vi "DB Update.vi"(8 "error in (no error)":errorcluster, 10 "SQL query":string, 11 "Database in":refnum<class "MYSQL Database.lvclass">) -> (0 "error out":errorcluster, 3 "Database out":refnum<class "MYSQL Database.lvclass">)   [LabVIEW 2023, in "HardwareAbstractionLayer_LVOOP.lvlib" / "MYSQL Database.lvclass"]
uses:
  MYSQL Database.lvclass
  MYSQL Database.lvclass/MYSQL Database.ctl
  <vilib>/addons/database/Connection.llb/Conn Execute.vi
  <vilib>/addons/database/Recordset.llb/Rec Destroy - Connection.vi
  <vilib>/addons/database/NI_Database_API.lvlib
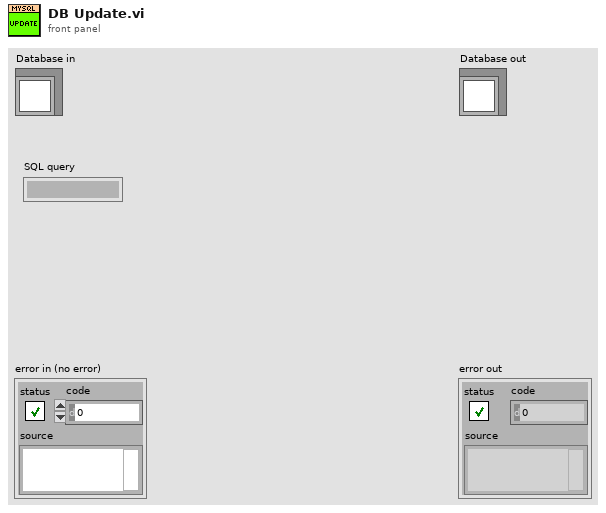
[diagram p1: front panel]
types:
  T1 = typedef "NI_Database_API.lvlib/Conn ObjectReference.ctl" = refnum<k1>
  T2 = typedef "NI_Database_API.lvlib/Rec ObjectReference.ctl" = refnum<k1>
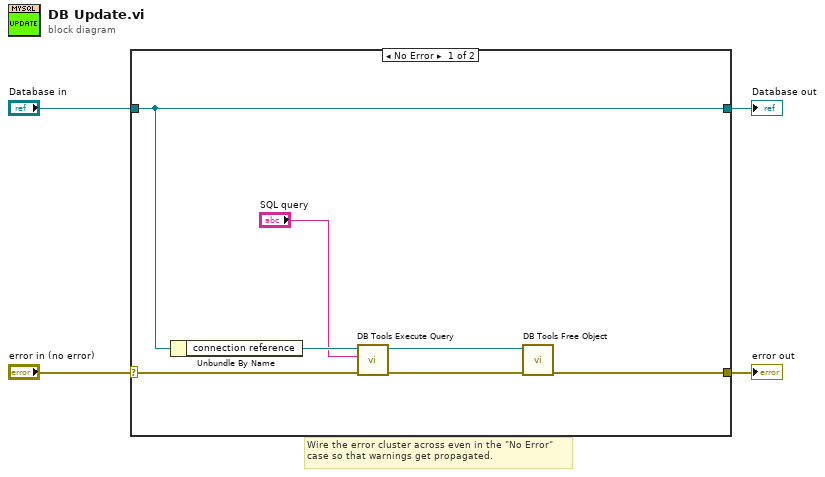
[diagram p0: block diagram]
diagram:
  # "Wire the error cluster across even in the \"No Error\"\ncase so that warnings get propagated."
  n1 = case shown="No Error" "error in (no error)" {
    selector: "error in (no error)" -> [w9 w13]
    tunnel: [w8 w13] -> w3
    tunnel: [w7 w12] -> w1
    tunnel: "Database in" -> [w7 w12]
    frame No Error {
      n2 = Unbundle By Name(w7) -> ("connection reference"=w6:T1)
      n3 = call-poly <vilib>:"DB Tools Execute Query.vi"("error in (no error)"=w9, "SQL query"="SQL query", "connection reference"=w6) -> ("error out"=w10:errorcluster, "recordset reference"=w11:T2)  [unwired: 5 in]
      n4 = call-poly <vilib>:"DB Tools Free Object.vi"("error in (no error)"=w10, "recordset reference"=w11) -> ("error out"=w8:errorcluster)  [unwired: 8 in, 1 out]
    }
    frame Error {
    }
  }
  "error out" <- w3
  "Database out" <- w1
